vi "unset metadata property.vi"(8 "error in":errorcluster, 10 "key":string, 11 "CEF_Configuration in":refnum<class "CEF_serializable configuration.lvclass">) -> (0 "error out":errorcluster, 3 "CEF_Configuration out":refnum<class "CEF_serializable configuration.lvclass">)   [LabVIEW 2023, in "CEF.lvlib" / "CEF_serializable configuration.lvclass"]
doc: "Clears a key/value pair stored in the configuration object.Copyright 2017 National Instruments Corporation\n\nLicensed under the Apache License, Version 2.0 (the \"License\"); you may not use this file except in compliance with the License. You may obtain a copy of the License at http://www.apache.org/licenses/LICENSE-2.0\nUnless required by applicable law or agreed to in writing, software distributed under the License is distributed on an \"AS IS\" BASIS, WITHOUT WARRANTIES OR CONDITIONS OF ANY KIND, either express or implied. See the License for the specific language governing permissions and limitations under the License."
uses:
  CEF_serializable configuration.lvclass
  CEF_serializable configuration.lvclass/CEF_serializable configuration.ctl
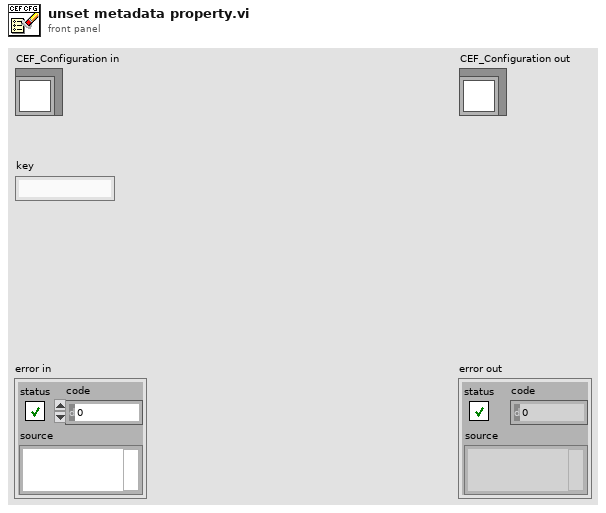
[diagram p1: front panel]
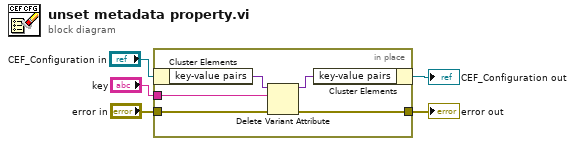
[diagram p0: block diagram]
diagram:
  n1 = in-place {
    in-place-border: "key" -> [w7]
    in-place-border: "error in" -> [w6]
    in-place-border: [w10] -> w1
    n2 = in-place-cluster #1("CEF_Configuration in") -> ("key-value pairs"=w8:variant)
    n3 = Delete Variant Attribute(4:w6, 6:w7, 7:w8) -> (0:w10:errorcluster, 3:w9:variant)  [unwired: 1 out]
    n4 = in-place-cluster #1("key-value pairs"=w9) -> (→"CEF_Configuration out":refnum<class "CEF_serializable configuration.lvclass">)
  }
  "error out" <- w1
